vi "LM Two H-Connected Asymmetric Gaussians and gradient.vi"(3 "output control":T1, 4 "data":variant, 5 "X":dbl[](array[numeric]), 6 "a":dbl[](array[numeric])) -> (0 "error out":errorcluster, 1 "f'(X,a)":dbl[][](array[numeric]), 2 "f(X,a)":dbl[](array[numeric]))   [LabVIEW 2021, in "Fits.lvlib"]
doc: "This template is the starting point for creating a model function to be passed to the Nonlinear Curve Fit.vi."
uses:
  Fits.lvlib
  <vilib>/gmath/NumericalOptimization/LM_output select.ctl
  D-Only Fixed Parameters.ctl
  <vilib>/gmath/NI_Gmath.lvlib
panel:
  # "Parameters:\n\namplitude 1: A1\ncenter 1: t1\nSDV 1-: s1-\nSDV 1+: s1+\nAmplitude 2: A2\ncenter 2: t2\nSDV 2-: s2-\nSDV 2+: s2+\nBridge Amplitude: A3"
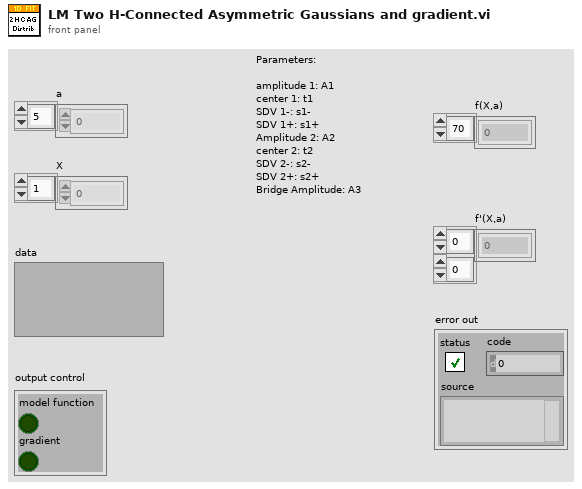
[diagram p1: front panel]
types:
  T1 = typedef "NI_Gmath.lvlib/LM_output select.ctl" = cluster{"model function":bool, "gradient":bool}
  T2 = typedef "Fits.lvlib/D-Only Fixed Parameters.ctl" = cluster{"Fix D-only Peak Location":bool, "Peak Location":dbl, "Fix D-only Peak FWHM":bool, "Peak FWHM":dbl}
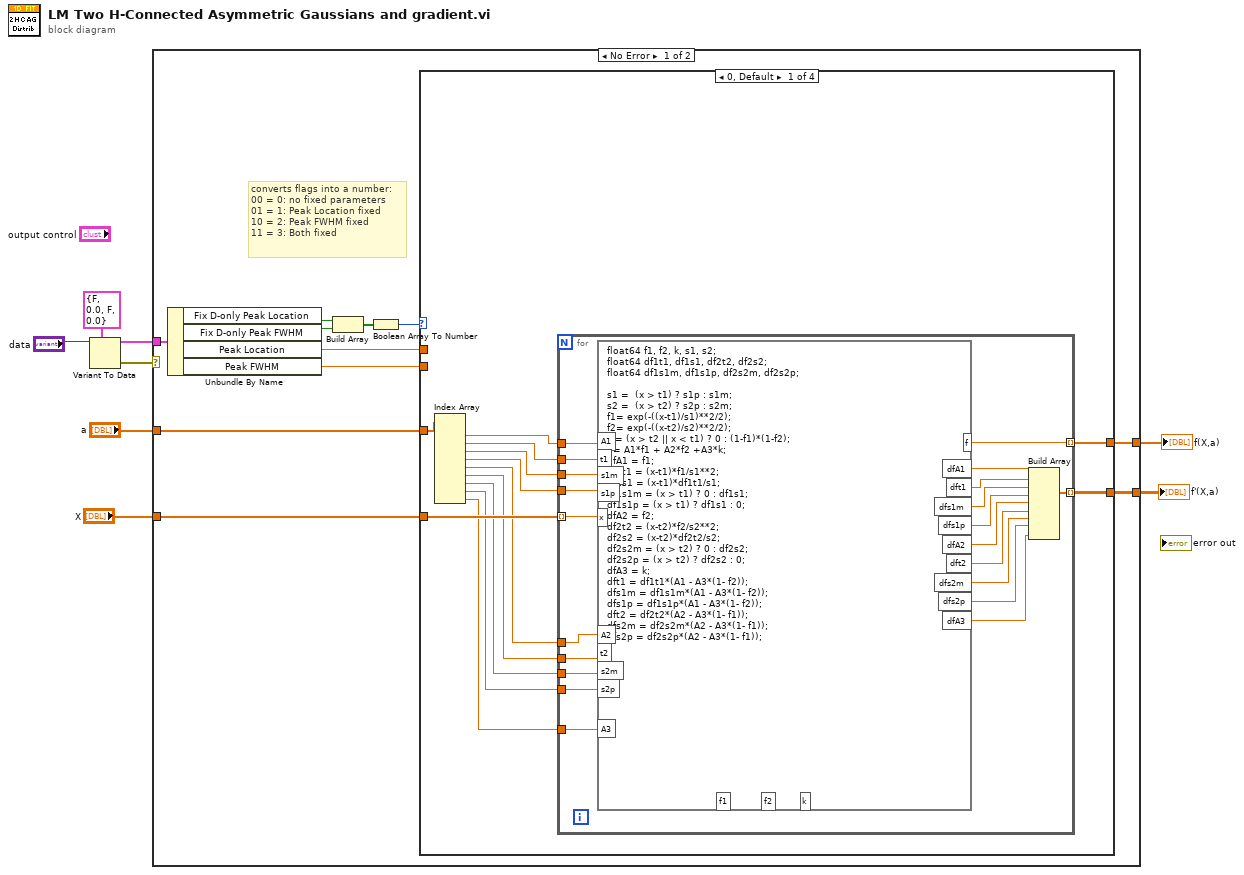
[diagram p0: block diagram]
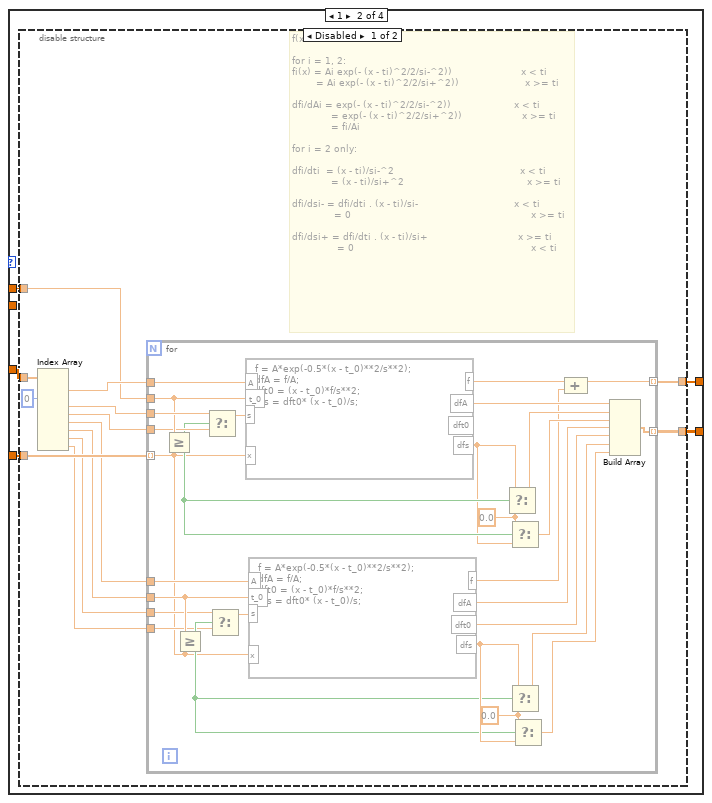
[diagram p2: hidden frame]
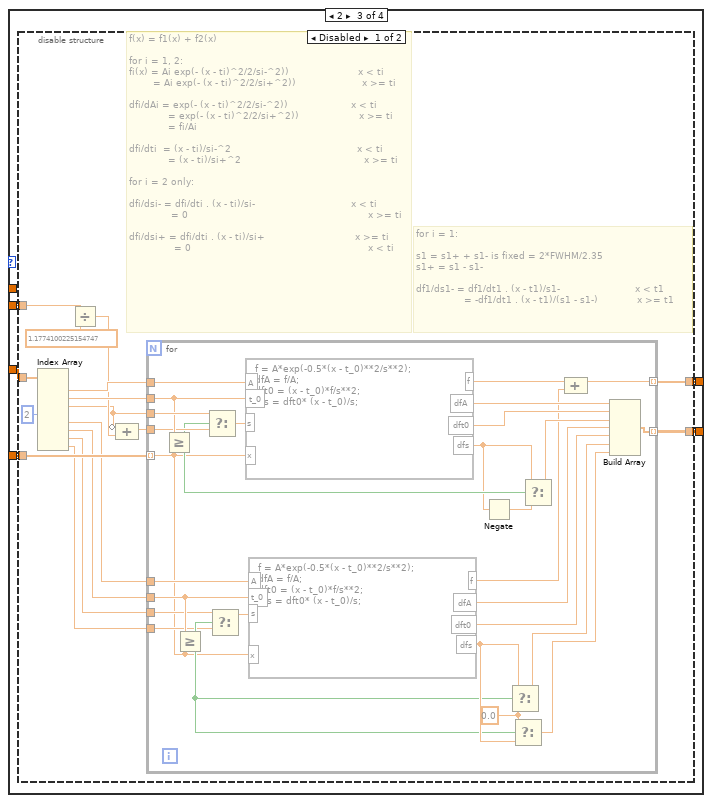
[diagram p4: hidden frame]
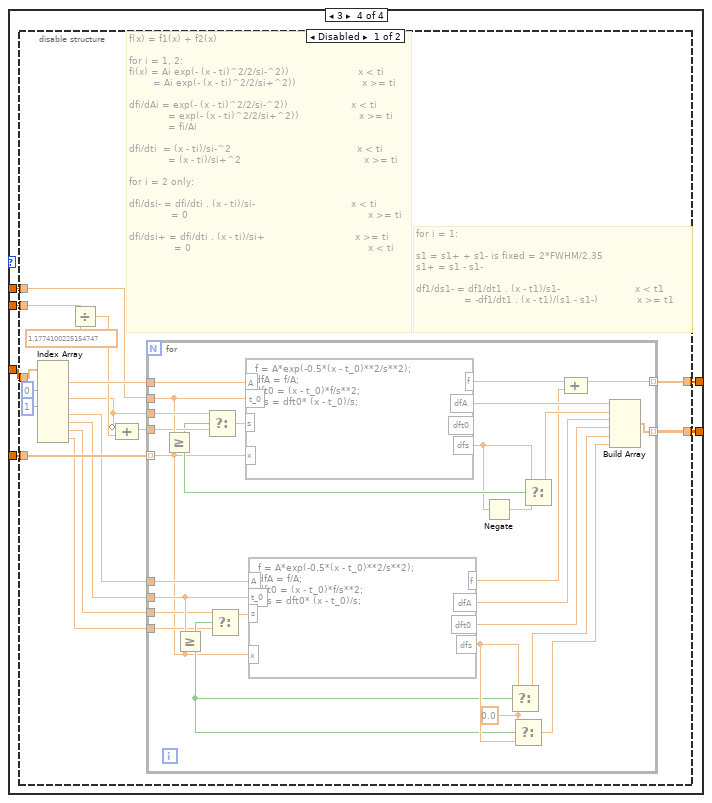
[diagram p6: hidden frame]
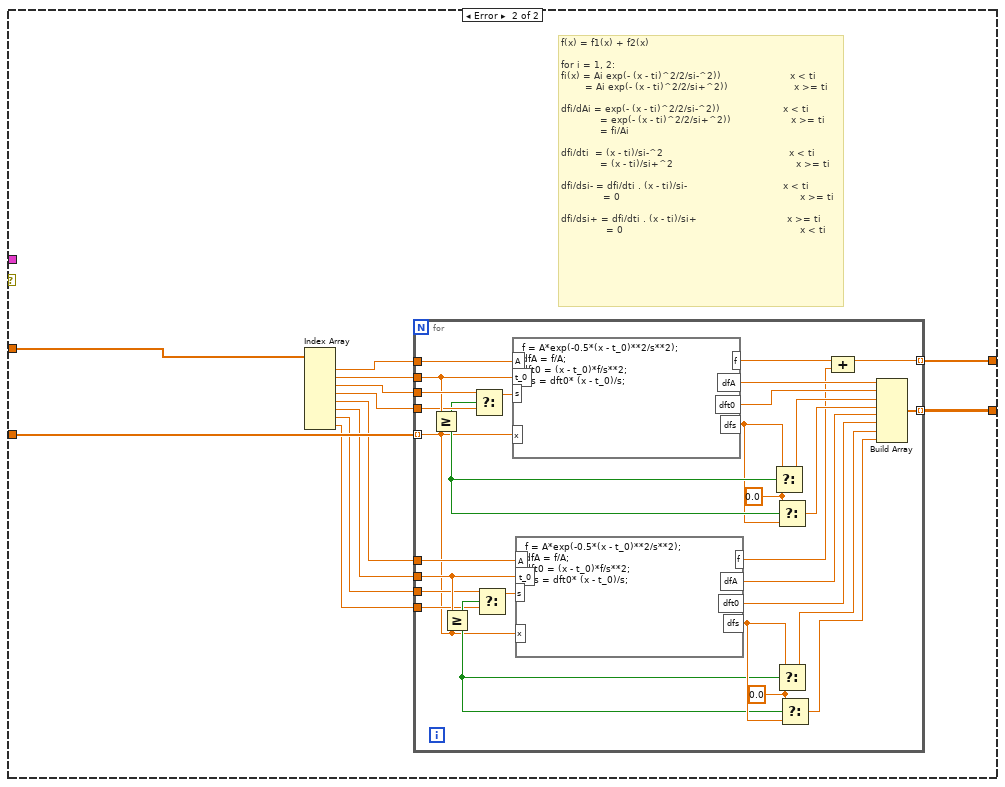
[diagram p8: hidden frame]
diagram:
  n1 = Variant To Data(type=T2 {"Fix D-only Peak Location"=FALSE, "Peak Location"=0.0, "Fix D-only Peak FWHM"=FALSE, "Peak FWHM"=0.0} ("Fixed Parameters"), Variant="data") -> (data=w1:T2, error out=w2:errorcluster)  [unwired: 1 in]
  n2 = case shown="No Error" w2 {
    tunnel: "a" -> [w19 w210]
    tunnel: "X" -> [w18 w205]
    tunnel: [w17 w200] -> w6
    tunnel: [w16 w199] -> w5
    tunnel: w1 -> [w12 _]
    frame No Error {
      # "converts flags into a number:\n00 = 0: no fixed parameters\n01 = 1: Peak Location fixed\n10 = 2: Peak FWHM fixed\n11 = 3: Both fixed"
      n3 = Unbundle By Name(w12) -> ("Fix D-only Peak Location"=w15:bool, "Fix D-only Peak FWHM"=w14:bool, "Peak Location"=w10:dbl, "Peak FWHM"=w9:dbl)
      n4 = Build Array(w15, w14) -> (w13:bool[])
      n5 = Boolean Array To Number(Boolean array=w13) -> (number=w11:u32)
      n6 = case shown="0, Default" w11 {
        tunnel: w19 -> [w32 w58 w104 w154]
        tunnel: w18 -> [w27 w57 w103 w153]
        tunnel: [w21 w56 w102 w152] -> w17
        tunnel: [w20 w55 w101 w151] -> w16
        tunnel: w10 -> [_ w54 _ w149]
        tunnel: w9 -> [_ _ w100 w150]
        frame 0, Default {
          n7 = Index Array(array=w32) -> (element #1=w31:dbl, element #2=w30:dbl, element #3=w29:dbl, element #4=w28:dbl, element #5=w26:dbl, element #6=w25:dbl, element #7=w24:dbl, element #8=w23:dbl, element #9=w22:dbl)  [unwired: 9 in]
          n8 = for {
            tunnel: w31 -> [w45]
            tunnel: w30 -> [w46]
            tunnel: w29 -> [w47]
            tunnel: w28 -> [w48]
            tunnel: w27 -> [w44] mode=indexing
            tunnel: w26 -> [w49]
            tunnel: w25 -> [w50]
            tunnel: w24 -> [w51]
            tunnel: w23 -> [w52]
            tunnel: w22 -> [w53]
            tunnel: [w43] -> w21 mode=indexing
            tunnel: [w33] -> w20 mode=indexing
            n9 = formula code="float64 f1, f2, k, s1, s2;\nfloat64 df1t1, df1s1, df2t2, df2s2;\nfloat64 df1s1m, df1s1p, df2s2m, df2s2p;\n\ns1 =  (x > t1) ? s1p : s1m;\ns2 =  (x > t2) ? s2p : s2m;\nf1= exp(-((x-t1)/s1)**2/2);\nf2= exp(-((x-t2)/s2)**2/2);\nk = (x > t2 || x < t1) ? 0 : (1-f1)*(1-f2);\nf = A1*f1 + A2*f2 +A3*k;\ndfA1 = f1;\ndf1t1 = (x-t1)*f1/s1**2;\ndf1s1 = (x-t1)*df1t1/s1;\ndf1s1m = (x > t1) ? 0 : df1s1;\ndf1s1p = (x > t1) ? df1s1 : 0;\ndfA2 = f2;\ndf2t2 = (x-t2)*f2/s2**2;\ndf2s2 = (x-t2)*df2t2/s2;\ndf2s2m = (x > t2) ? 0 : df2s2;\ndf2s2p = (x > t2) ? df2s2 : 0;\ndfA3 = k;\ndft1 = df1t1*(A1 - A3*(1- f2));\ndfs1m = df1s1m*(A1 - A3*(1- f2));\ndfs1p = df1s1p*(A1 - A3*(1- f2));\ndft2 = df2t2*(A2 - A3*(1- f1));\ndfs2m = df2s2m*(A2 - A3*(1- f1));\ndfs2p = df2s2p*(A2 - A3*(1- f1));"("A1"=w45, "t1"=w46, "s1m"=w47, "x"=w44, "A2"=w49, "t2"=w50, "s2m"=w51, "A3"=w53, "s1p"=w48, "s2p"=w52) -> ("f"=w43:dbl, "dfA1"=w42:dbl, "dft1"=w41:dbl, "dfs1m"=w40:dbl, "dfA2"=w38:dbl, "dft2"=w37:dbl, "dfs2m"=w36:dbl, "dfA3"=w34:dbl, "dfs1p"=w39:dbl, "dfs2p"=w35:dbl)  [unwired: 3 out]
            n10 = Build Array(w42, w41, w40, w39, w38, w37, w36, w35, w34) -> (w33:dbl[])
          }
        }
        frame 1 {
          n11 = disable-structure shown="Disabled" {
            disable-tunnel: w58 -> [w71 _]
            disable-tunnel: w57 -> [w67 _]
            disable-tunnel: [w62 _] -> w56
            disable-tunnel: [w61 _] -> w55
            disable-tunnel: w54 -> [w60 _]
            frame Disabled {
              # "f(x) = f1(x) + f2(x)\n\nfor i = 1, 2: \nfi(x) = Ai exp(- (x - ti)^2/2/si-^2))                       x < ti\n        = Ai exp(- (x - ti)^2/2/si+^2))                      x >= ti\n\ndfi/dAi = exp(- (x - ti)^2/2/si-^2))                     x < ti\n             = exp(- (x - ti)^2/2/si+^2))                    x >= ti\n             = fi/Ai\n\nfor i = 2 only: \n\ndfi/dti  = (x - ti)/si-^2                                          x < ti\n             = (x - ti)/si+^2                                         x >= ti\n\ndfi/dsi- = dfi/dti . (x - ti)/si-                                x < ti\n              = 0                                                            x >= ti\n\ndfi/dsi+ = dfi/dti . (x - ti)/si+                              x >= ti\n               = 0                                                           x < ti"
              n12 = Index Array(array=w71, index #2=0 ("index")) -> (element #1=w70:dbl, element #3=w69:dbl, element #4=w68:dbl, element #5=w66:dbl, element #6=w65:dbl, element #7=w64:dbl, element #8=w63:dbl)  [unwired: 7 in, 1 out]
              n13 = for {
                tunnel: w70 -> [w99]
                tunnel: w60 -> [w96]
                tunnel: w69 -> [w98]
                tunnel: w68 -> [w95]
                tunnel: w67 -> [w78] mode=indexing
                tunnel: [w77] -> w62 mode=indexing
                tunnel: [w87] -> w61 mode=indexing
                tunnel: w66 -> [w82]
                tunnel: w65 -> [w81]
                tunnel: w64 -> [w80]
                tunnel: w63 -> [w79]
                w85 = 0.0 ("f")
                w93 = 0.0 ("f")
                n14 = Greater Or Equal?(x=w96, y=w78) -> (x >= y?=w94:bool)
                n15 = Greater Or Equal?(x=w81, y=w78) -> (x >= y?=w84:bool)
                n16 = Select(t=w98, s=w94, f=w95) -> (s? t:f=w97:dbl)
                n17 = Select(t=w80, s=w84, f=w79) -> (s? t:f=w83:dbl)
                n18 = formula code="f = A*exp(-0.5*(x - t_0)**2/s**2);\ndfA = f/A;\ndft0 = (x - t_0)*f/s**2;\ndfs = dft0* (x - t_0)/s;"("A"=w99, "t_0"=w96, "s"=w97, "x"=w78) -> ("f"=w90:dbl, "dfA"=w91:dbl, "dfs"=w92:dbl)  [unwired: 1 out]
                n19 = formula code="f = A*exp(-0.5*(x - t_0)**2/s**2);\ndfA = f/A;\ndft0 = (x - t_0)*f/s**2;\ndfs = dft0* (x - t_0)/s;"("A"=w82, "t_0"=w81, "s"=w83, "x"=w78) -> ("f"=w76:dbl, "dfA"=w75:dbl, "dft0"=w74:dbl, "dfs"=w86:dbl)
                n20 = Select(t=w92, s=w94, f=w93) -> (s? t:f=w89:dbl)
                n21 = Select(t=w93, s=w94, f=w92) -> (s? t:f=w88:dbl)
                n22 = Select(t=w86, s=w84, f=w85) -> (s? t:f=w73:dbl)
                n23 = Select(t=w85, s=w84, f=w86) -> (s? t:f=w72:dbl)
                n24 = Compound Arithmetic op=ADD(w90, w76) -> (w77:dbl)
                n25 = Build Array(w91, w89, w88, w75, w74, w73, w72) -> (w87:dbl[])
              }
            }
            frame Enabled {
            }
          }
        }
        frame 2 {
          n26 = disable-structure shown="Disabled" {
            disable-tunnel: w104 -> [w120 _]
            disable-tunnel: w103 -> [w117 _]
            disable-tunnel: [w112 _] -> w102
            disable-tunnel: [w111 _] -> w101
            disable-tunnel: w100 -> [w110 _]
            frame Disabled {
              # "for i = 1: \n\ns1 = s1+ + s1- is fixed = 2*FWHM/2.35\ns1+ = s1 - s1-\n\ndf1/ds1- = df1/dt1 . (x - t1)/s1-                         x < t1\n                = -df1/dt1 . (x - t1)/(s1 - s1-)             x >= t1"
              # "f(x) = f1(x) + f2(x)\n\nfor i = 1, 2: \nfi(x) = Ai exp(- (x - ti)^2/2/si-^2))                       x < ti\n        = Ai exp(- (x - ti)^2/2/si+^2))                      x >= ti\n\ndfi/dAi = exp(- (x - ti)^2/2/si-^2))                     x < ti\n             = exp(- (x - ti)^2/2/si+^2))                    x >= ti\n             = fi/Ai\n\ndfi/dti  = (x - ti)/si-^2                                          x < ti\n             = (x - ti)/si+^2                                         x >= ti\n\nfor i = 2 only: \n\ndfi/dsi- = dfi/dti . (x - ti)/si-                                x < ti\n              = 0                                                            x >= ti\n\ndfi/dsi+ = dfi/dti . (x - ti)/si+                              x >= ti\n               = 0                                                           x < ti"
              n27 = Index Array(array=w120, index #4=2 ("index")) -> (element #1=w119:dbl, element #2=w118:dbl, element #3=w106:dbl, element #5=w116:dbl, element #6=w115:dbl, element #7=w114:dbl, element #8=w113:dbl)  [unwired: 7 in, 1 out]
              n28 = Divide(x=w110, y=1.1774100225154747) -> (x/y=w107:dbl)
              n29 = Compound Arithmetic op=ADD(invert w106, w107) -> (w105:dbl)
              n30 = for {
                tunnel: w119 -> [w148]
                tunnel: w118 -> [w145]
                tunnel: w106 -> [w147]
                tunnel: w105 -> [w144]
                tunnel: w117 -> [w129] mode=indexing
                tunnel: [w128] -> w112 mode=indexing
                tunnel: [w138] -> w111 mode=indexing
                tunnel: w116 -> [w133]
                tunnel: w115 -> [w132]
                tunnel: w114 -> [w131]
                tunnel: w113 -> [w130]
                w136 = 0.0 ("f")
                n31 = Greater Or Equal?(x=w145, y=w129) -> (x >= y?=w143:bool)
                n32 = Greater Or Equal?(x=w132, y=w129) -> (x >= y?=w135:bool)
                n33 = Select(t=w147, s=w143, f=w144) -> (s? t:f=w146:dbl)
                n34 = Select(t=w131, s=w135, f=w130) -> (s? t:f=w134:dbl)
                n35 = formula code="f = A*exp(-0.5*(x - t_0)**2/s**2);\ndfA = f/A;\ndft0 = (x - t_0)*f/s**2;\ndfs = dft0* (x - t_0)/s;"("A"=w148, "t_0"=w145, "s"=w146, "x"=w129) -> ("f"=w141:dbl, "dfA"=w142:dbl, "dft0"=w140:dbl, "dfs"=w122:dbl)
                n36 = formula code="f = A*exp(-0.5*(x - t_0)**2/s**2);\ndfA = f/A;\ndft0 = (x - t_0)*f/s**2;\ndfs = dft0* (x - t_0)/s;"("A"=w133, "t_0"=w132, "s"=w134, "x"=w129) -> ("f"=w127:dbl, "dfA"=w126:dbl, "dft0"=w125:dbl, "dfs"=w137:dbl)
                n37 = Negate(x=w122) -> (-x=w121:dbl)
                n38 = Select(t=w137, s=w135, f=w136) -> (s? t:f=w124:dbl)
                n39 = Select(t=w136, s=w135, f=w137) -> (s? t:f=w123:dbl)
                n40 = Select(t=w122, s=w143, f=w121) -> (s? t:f=w139:dbl)
                n41 = Compound Arithmetic op=ADD(w141, w127) -> (w128:dbl)
                n42 = Build Array(w142, w140, w139, w126, w125, w124, w123) -> (w138:dbl[])
              }
            }
            frame Enabled {
            }
          }
        }
        frame 3 {
          n43 = disable-structure shown="Disabled" {
            disable-tunnel: w154 -> [w171 _]
            disable-tunnel: w153 -> [w169 _]
            disable-tunnel: [w164 _] -> w152
            disable-tunnel: [w163 _] -> w151
            disable-tunnel: w150 -> [w162 _]
            disable-tunnel: w149 -> [w156 _]
            frame Disabled {
              # "for i = 1: \n\ns1 = s1+ + s1- is fixed = 2*FWHM/2.35\ns1+ = s1 - s1-\n\ndf1/ds1- = df1/dt1 . (x - t1)/s1-                         x < t1\n                = -df1/dt1 . (x - t1)/(s1 - s1-)             x >= t1"
              # "f(x) = f1(x) + f2(x)\n\nfor i = 1, 2: \nfi(x) = Ai exp(- (x - ti)^2/2/si-^2))                       x < ti\n        = Ai exp(- (x - ti)^2/2/si+^2))                      x >= ti\n\ndfi/dAi = exp(- (x - ti)^2/2/si-^2))                     x < ti\n             = exp(- (x - ti)^2/2/si+^2))                    x >= ti\n             = fi/Ai\n\ndfi/dti  = (x - ti)/si-^2                                          x < ti\n             = (x - ti)/si+^2                                         x >= ti\n\nfor i = 2 only: \n\ndfi/dsi- = dfi/dti . (x - ti)/si-                                x < ti\n              = 0                                                            x >= ti\n\ndfi/dsi+ = dfi/dti . (x - ti)/si+                              x >= ti\n               = 0                                                           x < ti"
              n44 = Index Array(array=w171, index #2=0 ("index"), index #4=1 ("index")) -> (element #1=w170:dbl, element #3=w158:dbl, element #5=w168:dbl, element #6=w167:dbl, element #7=w166:dbl, element #8=w165:dbl)  [unwired: 6 in, 2 out]
              n45 = Divide(x=w162, y=1.1774100225154747) -> (x/y=w159:dbl)
              n46 = Compound Arithmetic op=ADD(invert w158, w159) -> (w157:dbl)
              n47 = for {
                tunnel: w170 -> [w198]
                tunnel: w156 -> [w195]
                tunnel: w158 -> [w197]
                tunnel: w157 -> [w194]
                tunnel: w169 -> [w180] mode=indexing
                tunnel: [w179] -> w164 mode=indexing
                tunnel: [w189] -> w163 mode=indexing
                tunnel: w168 -> [w184]
                tunnel: w167 -> [w183]
                tunnel: w166 -> [w182]
                tunnel: w165 -> [w181]
                w187 = 0.0 ("f")
                n48 = Greater Or Equal?(x=w195, y=w180) -> (x >= y?=w193:bool)
                n49 = Greater Or Equal?(x=w183, y=w180) -> (x >= y?=w186:bool)
                n50 = Select(t=w197, s=w193, f=w194) -> (s? t:f=w196:dbl)
                n51 = Select(t=w182, s=w186, f=w181) -> (s? t:f=w185:dbl)
                n52 = formula code="f = A*exp(-0.5*(x - t_0)**2/s**2);\ndfA = f/A;\ndft0 = (x - t_0)*f/s**2;\ndfs = dft0* (x - t_0)/s;"("A"=w198, "t_0"=w195, "s"=w196, "x"=w180) -> ("f"=w191:dbl, "dfA"=w192:dbl, "dfs"=w173:dbl)  [unwired: 1 out]
                n53 = formula code="f = A*exp(-0.5*(x - t_0)**2/s**2);\ndfA = f/A;\ndft0 = (x - t_0)*f/s**2;\ndfs = dft0* (x - t_0)/s;"("A"=w184, "t_0"=w183, "s"=w185, "x"=w180) -> ("f"=w178:dbl, "dfA"=w177:dbl, "dft0"=w176:dbl, "dfs"=w188:dbl)
                n54 = Negate(x=w173) -> (-x=w172:dbl)
                n55 = Select(t=w188, s=w186, f=w187) -> (s? t:f=w175:dbl)
                n56 = Select(t=w187, s=w186, f=w188) -> (s? t:f=w174:dbl)
                n57 = Select(t=w173, s=w193, f=w172) -> (s? t:f=w190:dbl)
                n58 = Compound Arithmetic op=ADD(w191, w178) -> (w179:dbl)
                n59 = Build Array(w192, w190, w177, w176, w175, w174) -> (w189:dbl[])
              }
            }
            frame Enabled {
            }
          }
        }
      }
    }
    frame Error {
      # "f(x) = f1(x) + f2(x)\n\nfor i = 1, 2: \nfi(x) = Ai exp(- (x - ti)^2/2/si-^2))                       x < ti\n        = Ai exp(- (x - ti)^2/2/si+^2))                      x >= ti\n\ndfi/dAi = exp(- (x - ti)^2/2/si-^2))                     x < ti\n             = exp(- (x - ti)^2/2/si+^2))                    x >= ti\n             = fi/Ai\n\ndfi/dti  = (x - ti)/si-^2                                          x < ti\n             = (x - ti)/si+^2                                         x >= ti\n\ndfi/dsi- = dfi/dti . (x - ti)/si-                                x < ti\n              = 0                                                            x >= ti\n\ndfi/dsi+ = dfi/dti . (x - ti)/si+                              x >= ti\n               = 0                                                           x < ti"
      n60 = Index Array(array=w210) -> (element #1=w209:dbl, element #2=w208:dbl, element #3=w207:dbl, element #4=w206:dbl, element #5=w204:dbl, element #6=w203:dbl, element #7=w202:dbl, element #8=w201:dbl)  [unwired: 8 in]
      n61 = for {
        tunnel: w209 -> [w239]
        tunnel: w208 -> [w236]
        tunnel: w207 -> [w238]
        tunnel: w206 -> [w235]
        tunnel: w205 -> [w217] mode=indexing
        tunnel: [w216] -> w200 mode=indexing
        tunnel: [w226] -> w199 mode=indexing
        tunnel: w204 -> [w221]
        tunnel: w203 -> [w220]
        tunnel: w202 -> [w219]
        tunnel: w201 -> [w218]
        w224 = 0.0 ("f")
        w233 = 0.0 ("f")
        n62 = Greater Or Equal?(x=w236, y=w217) -> (x >= y?=w234:bool)
        n63 = Greater Or Equal?(x=w220, y=w217) -> (x >= y?=w223:bool)
        n64 = Select(t=w238, s=w234, f=w235) -> (s? t:f=w237:dbl)
        n65 = Select(t=w219, s=w223, f=w218) -> (s? t:f=w222:dbl)
        n66 = formula code="f = A*exp(-0.5*(x - t_0)**2/s**2);\ndfA = f/A;\ndft0 = (x - t_0)*f/s**2;\ndfs = dft0* (x - t_0)/s;"("A"=w239, "t_0"=w236, "s"=w237, "x"=w217) -> ("f"=w230:dbl, "dfA"=w231:dbl, "dft0"=w229:dbl, "dfs"=w232:dbl)
        n67 = formula code="f = A*exp(-0.5*(x - t_0)**2/s**2);\ndfA = f/A;\ndft0 = (x - t_0)*f/s**2;\ndfs = dft0* (x - t_0)/s;"("A"=w221, "t_0"=w220, "s"=w222, "x"=w217) -> ("f"=w215:dbl, "dfA"=w214:dbl, "dft0"=w213:dbl, "dfs"=w225:dbl)
        n68 = Select(t=w232, s=w234, f=w233) -> (s? t:f=w228:dbl)
        n69 = Select(t=w233, s=w234, f=w232) -> (s? t:f=w227:dbl)
        n70 = Select(t=w225, s=w223, f=w224) -> (s? t:f=w212:dbl)
        n71 = Select(t=w224, s=w223, f=w225) -> (s? t:f=w211:dbl)
        n72 = Compound Arithmetic op=ADD(w230, w215) -> (w216:dbl)
        n73 = Build Array(w231, w229, w228, w227, w214, w213, w212, w211) -> (w226:dbl[])
      }
    }
  }
  "f(X,a)" <- w6
  "f'(X,a)" <- w5
